vi "MagLab Hub Client.vi"() -> ()   [LabVIEW 2024]
uses:
  MagX/Add-on Storage.ctl
  MagX/Experiment info.ctl
panel:
  in  "Append to Wiki":bool
  in  "Create Markdown":bool
  in  "Upload file":bool
  in  "Logoff":bool
  out "Experiment info":T1
  out "Principal Investigator":string
  in  "Change experiment":bool
  in  "Logon":bool
  in  "Add-on storage":T2
  out "Experiment":string
  out "OSF user":string
  out "Experiment title":string="Undocumented activity"
  out "Project title":string="Undocumented activity"
  in  "File prefix":string="_c1_"
  in  "Computer":string="magdaq1"
  in  "Hub address":string="magfair.lanl.gov"
  in  "Station":string="Cell_1"
  in  "Stop Button":bool
  # "OSF Syncronization"
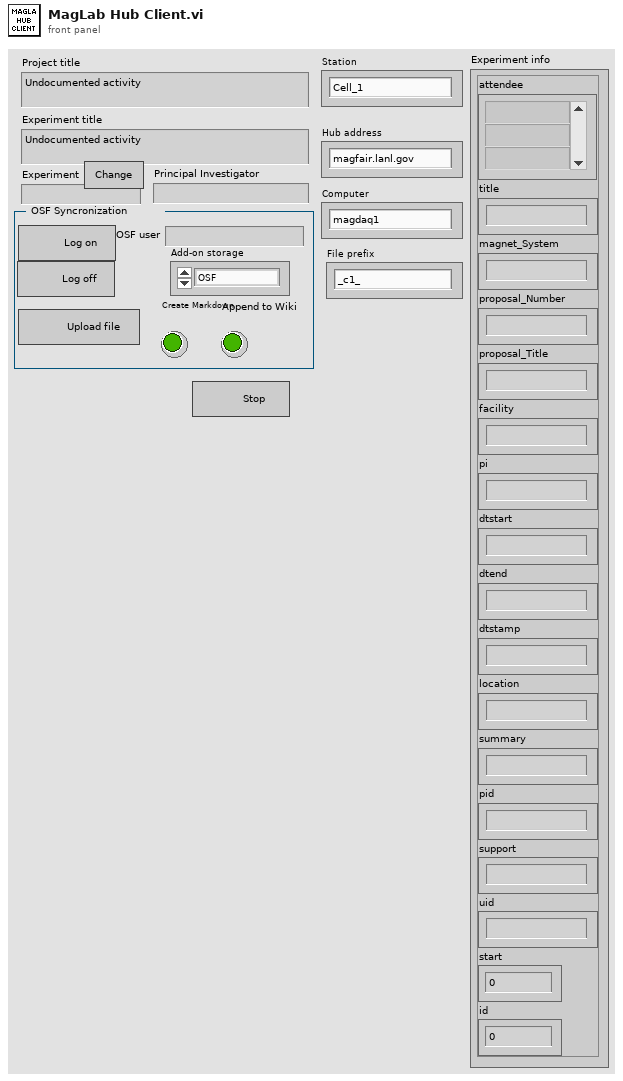
[diagram p1: front panel]
types:
  T1 = typedef "Experiment info.ctl" = cluster{"attendee":string[], "title":string, "magnet_System":string, "proposal_Number":string, "proposal_Title":string, "facility":string, "pi":string, "dtstart":string, "dtend":string, "dtstamp":string, "location":string, "summary":string, "pid":string, "support":string, "uid":string, "start":u64, "id":u64}
  T2 = typedef "Add-on Storage.ctl" = enum16{"OSF", "OSF - Split", "Google Drive", "Dropbox", "Box"}
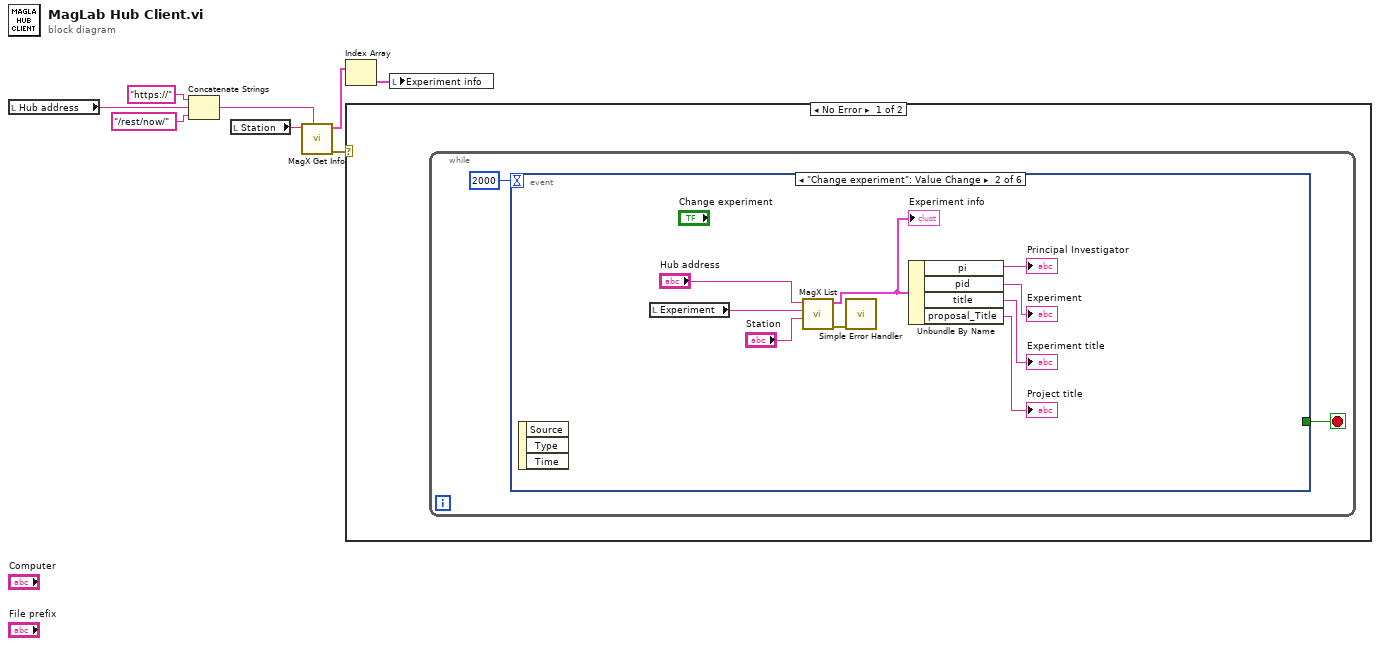
[diagram p0: block diagram]
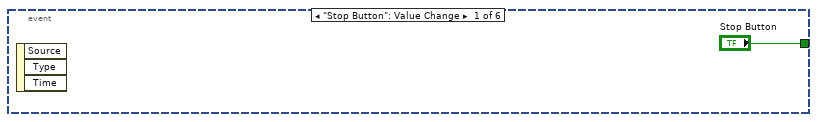
[diagram p2: hidden frame]
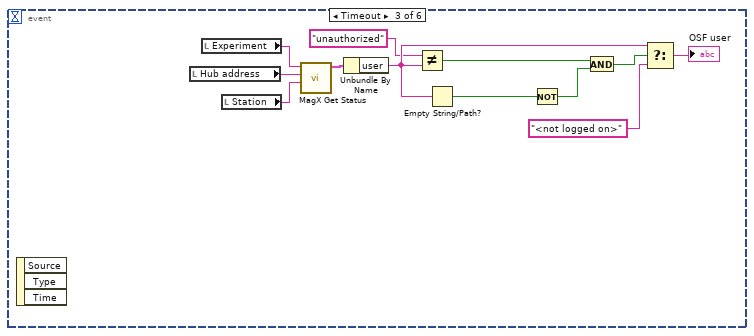
[diagram p3: hidden frame]
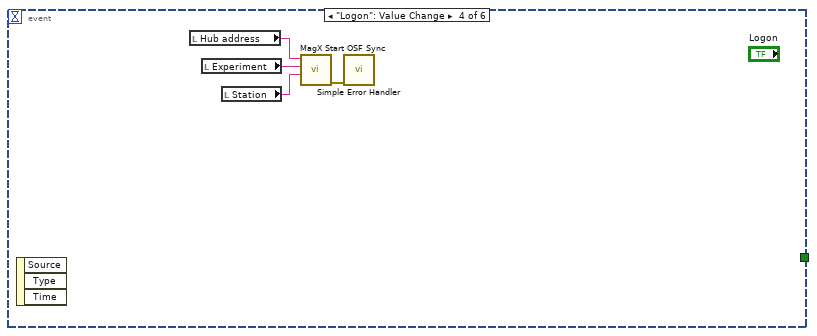
[diagram p4: hidden frame]
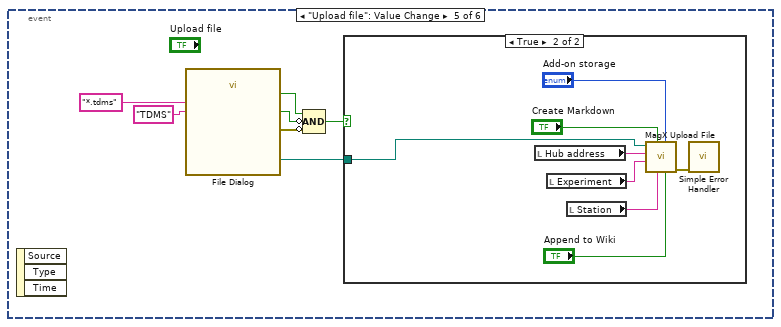
[diagram p5: hidden frame]
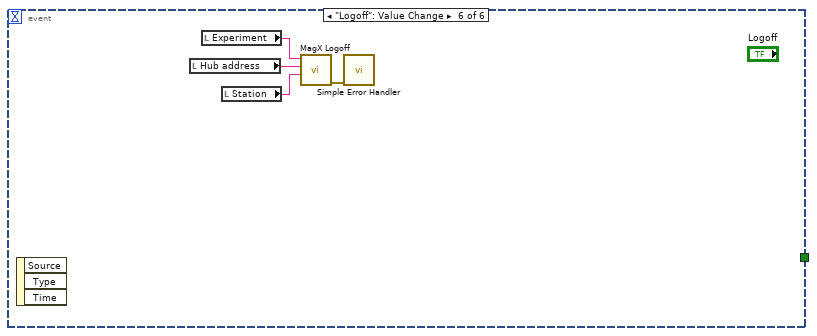
[diagram p7: hidden frame]
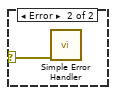
[diagram p8: hidden frame]
diagram:
  n1 = local read "Hub address"() -> (w2:string)
  n2 = Concatenate Strings("https://" ("string"), w2, "/rest/now/" ("string")) -> (w1:string)
  n3 = local read "Station"() -> (w7:string)
  n4 = call "MagX Get Info.vi"("url"=w1, "Station"=w7) -> ("error out"=w8:errorcluster, "Data out"=w6:T1[])  [unwired: 7 in, 1 out]
  n5 = Index Array(array=w6) -> (element=w5:T1)  [unwired: 1 in]
  n6 = case shown="No Error" w8 {
    selector: w8 -> [_ w56]
    frame No Error {
      n7 = while {
        stop <- w10 stop-if-true
        n8 = event shown="[1] \"Change experiment\": Value Change" {
          selector: _ -> [_ _ _ _ _ _]
          dyn-events: _ -> [_ _ _ _ _ _]
          timeout: 2000 -> [_ _ _ _ _ _]
          tunnel: ["Stop Button" _ _ _ _ _] -> w10
          event "Stop Button": Value Change {
            n9 = event-data() -> ()  [unwired: 1 in, 3 out]
          }
          event "Change experiment": Value Change {
            n10 = event-data() -> ()  [unwired: 1 in, 3 out]
            n11 = local read "Experiment"() -> (w20:string)
            n12 = call "MagX List.vi"("Current station in"="Station", "Initial Selection"=w20, "Hub URL"="Hub address") -> ("error out"=w12:errorcluster, "Experiment info"=w18:T1)  [unwired: 5 in, 2 out]
            "Experiment info" <- w18
            n13 = call <vilib>:"Simple Error Handler.vi"("error in (no error)"=w12) -> ()  [unwired: 4 in, 5 out]
            n14 = Unbundle By Name(w18) -> ("pi"=→"Principal Investigator":string, "pid"=→"Experiment":string, "title"=→"Experiment title":string, "proposal_Title"=→"Project title":string)
          }
          event Timeout {
            n15 = event-data() -> ()  [unwired: 1 in, 3 out]
            n16 = local read "Hub address"() -> (w31:string)
            n17 = local read "Experiment"() -> (w32:string)
            n18 = local read "Station"() -> (w30:string)
            n19 = call "MagX Get Status.vi"("Station"=w30, "MagLab OSF tool server"=w31, "Experiment ID"=w32) -> ("Data out"=w23:cluster{"user":string, "expid":string})  [unwired: 7 in, 1 out]
            n20 = Unbundle By Name(w23) -> ("user"=w28:string)
            n21 = Not Equal?(x="unauthorized" ("Control Name"), y=w28) -> (x != y?=w26:bool)
            n22 = Empty String/Path?(string/path=w28) -> (empty?=w25:bool)
            n23 = Not(x=w25) -> (.not. x?=w29:bool)
            n24 = And(x=w26, y=w29) -> (x .and. y?=w22:bool)
            n25 = Select(t=w28, s=w22, f="<not logged on>" ("Control Name")) -> (s? t:f=→"OSF user":string)
          }
          event "Logon": Value Change {
            n26 = event-data() -> ()  [unwired: 1 in, 3 out]
            n27 = local read "Hub address"() -> (w36:string)
            n28 = local read "Experiment"() -> (w35:string)
            n29 = local read "Station"() -> (w34:string)
            n30 = call "MagX Start OSF Sync.vi"("Station"=w34, "Experiment ID"=w35, "MagLab OSF tool server"=w36) -> ("error out"=w33:errorcluster)  [unwired: 8 in]
            n31 = call <vilib>:"Simple Error Handler.vi"("error in (no error)"=w33) -> ()  [unwired: 4 in, 5 out]
          }
          event "Upload file": Value Change {
            n32 = event-data() -> ()  [unwired: 1 in, 3 out]
            n33 = call "File Dialog"("pattern (all files)"="*.tdms", "pattern label"="TDMS") -> ("selected path"=w37:path, "exists"=w41:bool, "cancelled"=w40:bool, "error out"=w39:errorcluster)  [unwired: 10 in]
            n34 = Compound Arithmetic op=AND(w41, invert w40, invert w39) -> (w38:bool)
            n35 = case shown="True" w38 {
              tunnel: w37 -> [_ w51]
              frame False {
              }
              frame True {
                n36 = local read "Hub address"() -> (w50:string)
                n37 = local read "Experiment"() -> (w49:string)
                n38 = local read "Station"() -> (w47:string)
                n39 = call "MagX Upload File.vi"("Append to Wiki"="Append to Wiki", "Add-on storage"="Add-on storage", "Station"=w47, "Create Markdown"="Create Markdown", "Experiment ID"=w49, "Log server"=w50, "File name"=w51) -> ("error out"=w48:errorcluster)  [unwired: 4 in]
                n40 = call <vilib>:"Simple Error Handler.vi"("error in (no error)"=w48) -> ()  [unwired: 4 in, 5 out]
              }
            }
          }
          event "Logoff": Value Change {
            n41 = event-data() -> ()  [unwired: 1 in, 3 out]
            n42 = local read "Hub address"() -> (w54:string)
            n43 = local read "Experiment"() -> (w55:string)
            n44 = local read "Station"() -> (w53:string)
            n45 = call "MagX Logoff.vi"("Station"=w53, "MagLab OSF tool server"=w54, "Experiment ID"=w55) -> ("error out"=w52:errorcluster)  [unwired: 8 in]
            n46 = call <vilib>:"Simple Error Handler.vi"("error in (no error)"=w52) -> ()  [unwired: 4 in, 5 out]
          }
        }
      }
    }
    frame Error {
      n47 = call <vilib>:"Simple Error Handler.vi"("error in (no error)"=w56) -> ()  [unwired: 4 in, 5 out]
    }
  }
  n48 = local write "Experiment info"(w5) -> ()
